vi "Limits Facade.vi"(0 "Data In":T7, 2 "Display State In":T2, 3 "Container State":T6) -> (6 "Data Out":T7, 7 "Display State Out":T2, 8 "Action":T1)   [LabVIEW 2013, in "Limits X.xctl"]
uses:
  Limits X.xctl
  Limits Data.ctl
  <vilib>/_xctls/Container State.ctl
  Limits State.ctl
  lib/Data Access Objects/Limits/DofTypes.ctl
  lib/Limits/Limite State.ctl
  lib/Apps/Yes No Button.ctl
  <vilib>/_xctls/Action.ctl
  <vilib>/_xctls/XControlSupport.lvlib
panel:
  in  "Limit Window":cluster{"Lower":dbl, "Upper":dbl, "Actual":dbl} caption="X1"
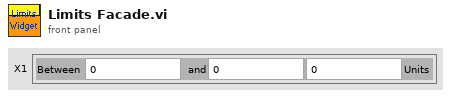
[diagram p1: front panel]
types:
  T1 = typedef "XControlSupport.lvlib/Action.ctl" = cluster{"Data Changed?":bool, "State Changed?":bool, "Action Name":string}
  T2 = typedef "Limits X.xctl/Limits State.ctl" = cluster{"DofType":T3, "Limit State":T4, "DOF Index":i32, "System Fault ":T5, "Has Lower":T5}
  T3 = typedef "DofTypes.ctl" = enum16{"Cartesian Displacements", "Cartesian Forces & Moments", "Actuator Displacements", "Actuator Forces", "Cartesian Increments", "Actuator Increments"}
  T4 = typedef "Limite State.ctl" = enum16{"Good", "Lower Bound Fault", "Upper Bound Fault"}
  T5 = typedef "Yes No Button.ctl" = bool
  T6 = typedef "XControlSupport.lvlib/Container State.ctl" = cluster{"Indicator?":bool, "Run Mode?":bool, " Refnum":refnum<vi>}
  T7 = typedef "Limits X.xctl/Limits Data.ctl" = cluster{"Lower":dbl, "Upper":dbl, "Actual":dbl}
  T8 = enum8{"Enabled", "Disabled", "Disabled and Grayed Out"}
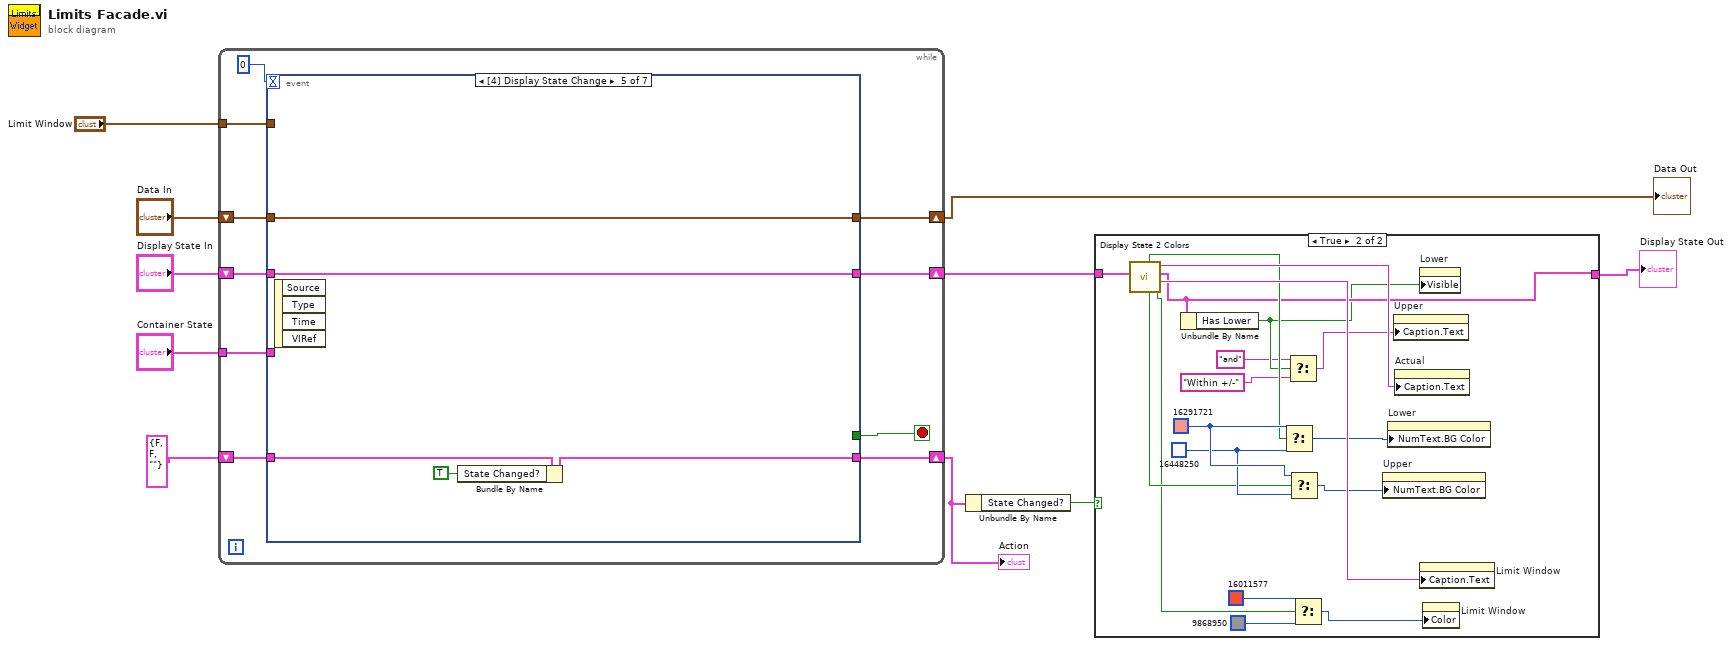
[diagram p0: block diagram]
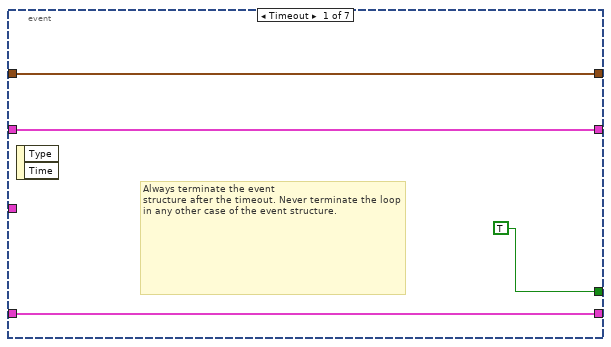
[diagram p3: hidden frame]
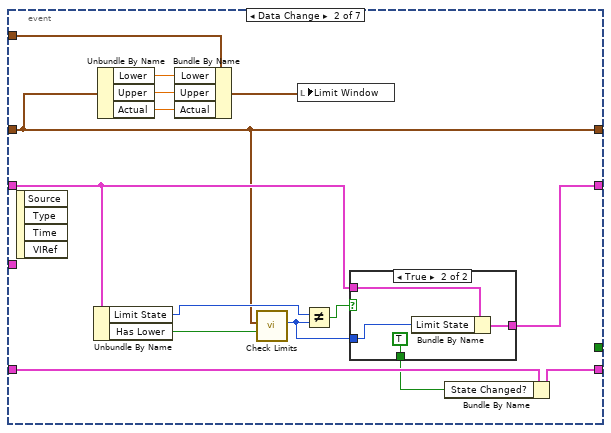
[diagram p4: hidden frame]
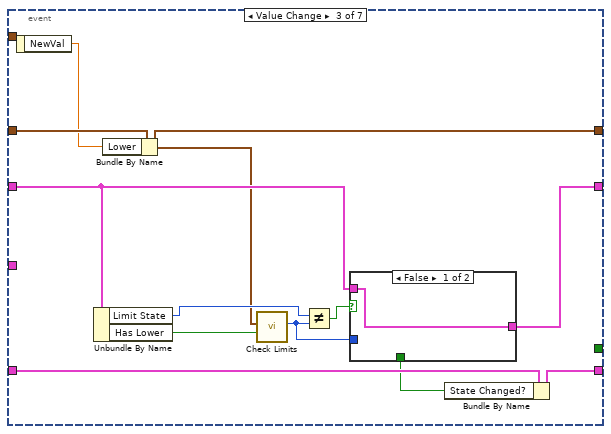
[diagram p6: hidden frame]
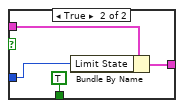
[diagram p7: hidden frame]
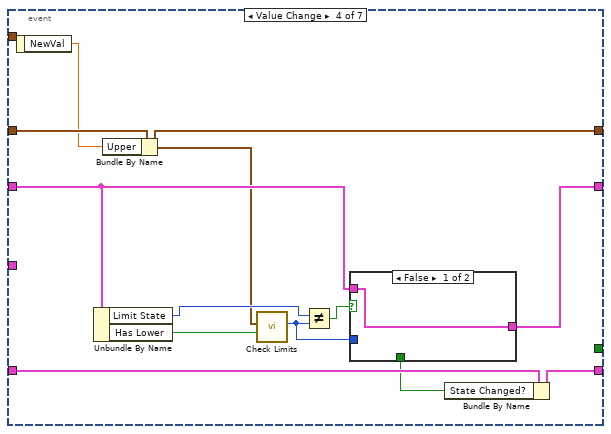
[diagram p8: hidden frame]
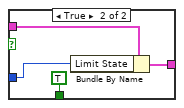
[diagram p9: hidden frame]
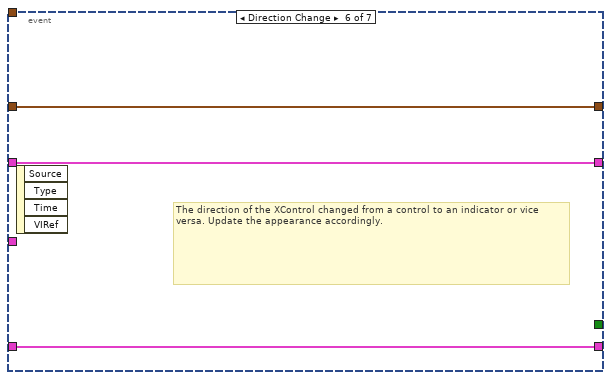
[diagram p10: hidden frame]
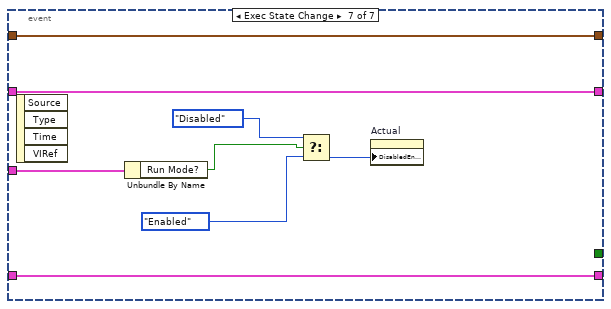
[diagram p11: hidden frame]
diagram:
  n1 = while {
    shift-right: [w19] -> w3
    shift-left: "Display State In" -> [w20]
    tunnel: "Container State" -> [w16]
    shift-right: [w14] -> w10
    shift-left: "Data In" -> [w15]
    shift-right: [w12] -> w5
    shift-left: T1 {"Data Changed?"=FALSE, "State Changed?"=FALSE, "Action Name"=""} ("Action") -> [w13]
    tunnel: "Limit Window" -> [w11]
    stop <- w18 stop-if-true
    n2 = event shown="[4] Display State Change" {
      selector: _ -> [_ _ _ _ _ _ _]
      dyn-events: _ -> [_ _ _ _ _ _ _]
      timeout: 0 -> [_ _ _ _ _ _ _]
      tunnel: w20 -> [w22 w31 w48 w65 w83 w86 w93]
      tunnel: [w22 w30 w47 w64 w83 w86 w93] -> w19
      tunnel: [TRUE _ _ _ _ _ _] -> w18
      tunnel: w16 -> [_ _ _ _ _ _ w94]
      tunnel: w15 -> [w21 w25 w55 w72 w82 w85 w92]
      tunnel: [w21 w25 w45 w62 w82 w85 w92] -> w14
      tunnel: [w23 w37 w54 w71 w80 w84 w91] -> w12
      tunnel: w13 -> [w23 w39 w56 w73 w81 w84 w91]
      tunnel: w11 -> [_ w29 _ _ _ _ _]
      event Timeout {
        # "Always terminate the event\nstructure after the timeout. Never terminate the loop in any other case of the event structure."
        n3 = event-data() -> ()  [unwired: 1 in, 2 out]
      }
      event Data Change {
        n4 = event-data() -> ()  [unwired: 1 in, 4 out]
        n5 = Unbundle By Name(w31) -> ("Limit State"=w35:T4, "Has Lower"=w36:T5)
        n6 = Unbundle By Name(w25) -> ("Lower"=w28:dbl, "Upper"=w27:dbl, "Actual"=w38:dbl)
        n7 = Bundle By Name(cluster=w29, "Lower"=w28, "Upper"=w27, "Actual"=w38) -> (w26:cluster{"Lower":dbl, "Upper":dbl, "Actual":dbl})
        n8 = call "Check Limits.vi"("Has Lower"=w36, "Limits Data"=w25) -> ("Limit State"=w33:T4)  [unwired: 9 in]
        n9 = local write "Limit Window"(w26) -> ()
        n10 = Not Equal?(x=w35, y=w33) -> (x != y?=w34:bool)
        n11 = case shown="True" w34 {
          tunnel: w33 -> [_ w43]
          tunnel: w31 -> [w40 w44]
          tunnel: [_ TRUE] -> w32
          tunnel: [w40 w41] -> w30
          frame False {
          }
          frame True {
            n12 = Bundle By Name(cluster=w44, "Limit State"=w43) -> (w41:T2)
          }
        }
        n13 = Bundle By Name(cluster=w39, "State Changed?"=w32) -> (w37:T1)
      }
      event "Limit Window.Lower": Value Change {
        n14 = event-data() -> ("NewVal"=w46:dbl)  [unwired: 1 in]
        n15 = Unbundle By Name(w48) -> ("Limit State"=w52:T4, "Has Lower"=w53:T5)
        n16 = Bundle By Name(cluster=w55, "Lower"=w46) -> (w45:T7)
        n17 = call "Check Limits.vi"("Has Lower"=w53, "Limits Data"=w45) -> ("Limit State"=w50:T4)  [unwired: 9 in]
        n18 = Not Equal?(x=w52, y=w50) -> (x != y?=w51:bool)
        n19 = case shown="False" w51 {
          tunnel: w50 -> [_ w60]
          tunnel: w48 -> [w57 w61]
          tunnel: [_ TRUE] -> w49
          tunnel: [w57 w58] -> w47
          frame False {
          }
          frame True {
            n20 = Bundle By Name(cluster=w61, "Limit State"=w60) -> (w58:T2)
          }
        }
        n21 = Bundle By Name(cluster=w56, "State Changed?"=w49) -> (w54:T1)
      }
      event "Limit Window.Upper": Value Change {
        n22 = event-data() -> ("NewVal"=w63:dbl)  [unwired: 1 in]
        n23 = Unbundle By Name(w65) -> ("Limit State"=w69:T4, "Has Lower"=w70:T5)
        n24 = Bundle By Name(cluster=w72, "Upper"=w63) -> (w62:T7)
        n25 = call "Check Limits.vi"("Has Lower"=w70, "Limits Data"=w62) -> ("Limit State"=w67:T4)  [unwired: 9 in]
        n26 = Not Equal?(x=w69, y=w67) -> (x != y?=w68:bool)
        n27 = case shown="False" w68 {
          tunnel: w67 -> [_ w77]
          tunnel: w65 -> [w74 w78]
          tunnel: [_ TRUE] -> w66
          tunnel: [w74 w75] -> w64
          frame False {
          }
          frame True {
            n28 = Bundle By Name(cluster=w78, "Limit State"=w77) -> (w75:T2)
          }
        }
        n29 = Bundle By Name(cluster=w73, "State Changed?"=w66) -> (w71:T1)
      }
      event Display State Change {
        n30 = event-data() -> ()  [unwired: 1 in, 4 out]
        n31 = Bundle By Name(cluster=w81, "State Changed?"=TRUE) -> (w80:T1)
      }
      event Direction Change {
        # "The direction of the XControl changed from a control to an indicator or vice versa. Update the appearance accordingly."
        n32 = event-data() -> ()  [unwired: 1 in, 4 out]
      }
      event Exec State Change {
        n33 = event-data() -> ()  [unwired: 1 in, 4 out]
        n34 = Unbundle By Name(w94) -> ("Run Mode?"=w88:bool)
        n35 = Select(t=T8."Disabled", s=w88, f=T8."Enabled" ("Disabled")) -> (s? t:f=w89:T8)
        n36 = property on="Actual" class="DigNum (strict)"("DisabledEnum"=w89) -> ()  [unwired: 2 in, 2 out]
      }
    }
  }
  "Data Out" <- w10
  "Action" <- w5
  n37 = Unbundle By Name(w5) -> ("State Changed?"=w4:bool)
  n38 = case shown="True" w4 {
    tunnel: w3 -> [w95 w113]
    tunnel: [w95 w100] -> w2
    frame False {
    }
    frame True {
      w109 = u32 16448250
      w110 = u32 16291721
      n39 = call "Display State 2 Colors.vi"("State In"=w113) -> ("Red BG"=w106:T5, "DOF Label"=w111:string, "State Out"=w100:T2, "Units"=w112:string, "Red Upper"=w107:T5, "Red Lower"=w108:T5)  [unwired: 5 in]
      n40 = Unbundle By Name(w100) -> ("Has Lower"=w99:T5)
      n41 = Select(t=w110, s=w108, f=w109) -> (s? t:f=w102:u32)
      n42 = Select(t="and" ("Caption.Text"), s=w99, f="Within +/-") -> (s? t:f=w97:string)
      n43 = Select(t=w110, s=w107, f=w109) -> (s? t:f=w101:u32)
      n44 = Select(t=u32 16011577, s=w106, f=u32 9868950) -> (s? t:f=w103:u32)
      n45 = property on="Upper" class="DigNum (strict)"("NumText.BG Color"=w101) -> ()  [unwired: 2 in, 2 out]
      n46 = property on="Lower" class="DigNum (strict)"("NumText.BG Color"=w102) -> ()  [unwired: 2 in, 2 out]
      n47 = property on="Upper" class="DigNum (strict)"("Caption.Text"=w97) -> ()  [unwired: 2 in, 2 out]
      n48 = property on="Actual" class="DigNum (strict)"("Caption.Text"=w112) -> ()  [unwired: 2 in, 2 out]
      n49 = property on="Lower" class="DigNum (strict)"("Visible"=w99) -> ()  [unwired: 2 in, 2 out]
      n50 = property on="Limit Window" class="Clust (strict)"("Caption.Text"=w111) -> ()  [unwired: 2 in, 2 out]
      n51 = property on="Limit Window" class="Clust (strict)"("Color"=w103) -> ()  [unwired: 2 in, 2 out]
    }
  }
  "Display State Out" <- w2
